vi "Get Intercept Point.vi"(8 "error in (no error)":errorcluster, 9 "Current  System of Reference Position":refnum<vi>, 10 "Tip Position":refnum<vi>, 11 "Angles":refnum<vi>) -> (0 "error out":errorcluster, 3 "Intercept Point":T1)   [LabVIEW 2012, in "Targeting Unit.lvlib"]
uses:
  Targeting Unit.lvlib
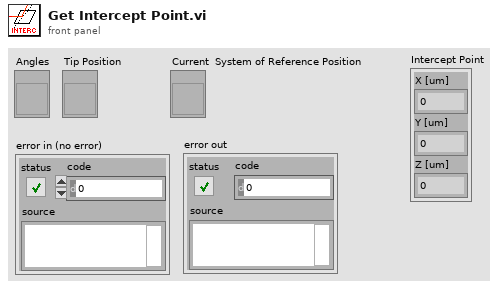
[diagram p1: front panel]
types:
  T1 = cluster{"X [um]":dbl, "Y [um]":dbl, "Z [um]":dbl}
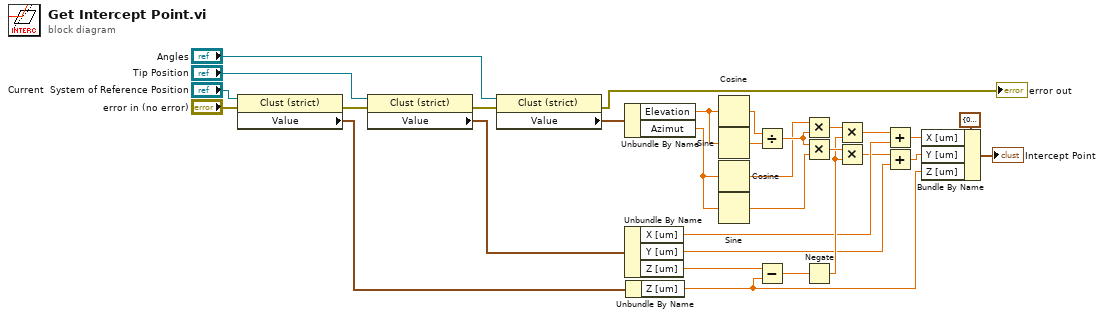
[diagram p0: block diagram]
diagram:
  n1 = property class="Clust (strict)"(reference="Current  System of Reference Position", error in="error in (no error)") -> (error out=w2:errorcluster, "Value"=w24:T1)  [unwired: 1 out]
  n2 = property class="Clust (strict)"(reference="Tip Position", error in=w2) -> (error out=w3:errorcluster, "Value"=w21:T1)  [unwired: 1 out]
  n3 = property class="Clust (strict)"(reference="Angles", error in=w3) -> (error out=→"error out":errorcluster, "Value"=w25:cluster{"Azimut":dbl, "Elevation":dbl})  [unwired: 1 out]
  n4 = Unbundle By Name(w25) -> ("Elevation"=w28:dbl, "Azimut"=w22:dbl)
  n5 = Unbundle By Name(w21) -> ("X [um]"=w7:dbl, "Y [um]"=w8:dbl, "Z [um]"=w9:dbl)
  n6 = Unbundle By Name(w24) -> ("Z [um]"=w10:dbl)
  n7 = Cosine(x=w28) -> (cos(x)=w29:dbl)
  n8 = Sine(x=w28) -> (sin(x)=w27:dbl)
  n9 = Cosine(x=w22) -> (cos(x)=w26:dbl)
  n10 = Sine(x=w22) -> (sin(x)=w23:dbl)
  n11 = Divide(x=w29, y=w27) -> (x/y=w30:dbl)
  n12 = Subtract(x=w9, y=w10) -> (x-y=w14:dbl)
  n13 = Multiply(x=w26, y=w30) -> (x*y=w13:dbl)
  n14 = Multiply(x=w30, y=w23) -> (x*y=w12:dbl)
  n15 = Negate(x=w14) -> (-x=w11:dbl)
  n16 = Multiply(x=w13, y=w11) -> (x*y=w6:dbl)
  n17 = Multiply(x=w12, y=w11) -> (x*y=w5:dbl)
  n18 = Add(x=w6, y=w7) -> (x+y=w16:dbl)
  n19 = Add(x=w5, y=w8) -> (x+y=w15:dbl)
  n20 = Bundle By Name(cluster=T1 {"X [um]"=0.0, "Y [um]"=0.0, "Z [um]"=0.0} ("y"), "X [um]"=w16, "Y [um]"=w15, "Z [um]"=w10) -> (→"Intercept Point":T1)
